vi "show_plot.vi"(6 "plot_id":i32, 8 "autoscale":bool, 9 "show_plot":bool, 11 "XYGraph Refnum":refnum<vi>) -> (0 "done":bool)   [LabVIEW 2025]
uses:
  305b2933-337f-4dbb-963a-25d37b027f8a.vi
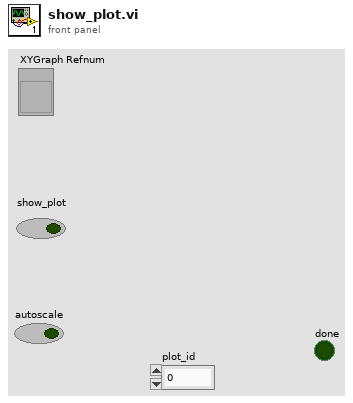
[diagram p1: front panel]
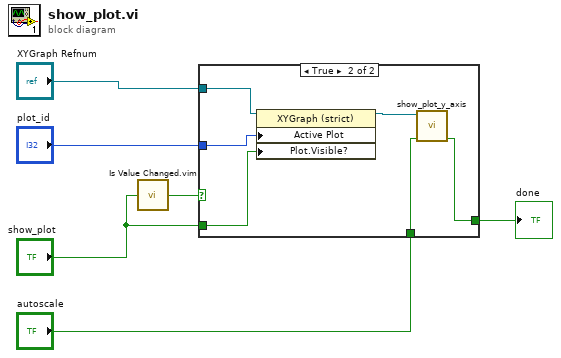
[diagram p0: block diagram]
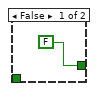
[diagram p2: hidden frame]
diagram:
  n1 = call "Is Value Changed.vim"("value"="show_plot") -> ("changed or first call?"=w6:bool)
  n2 = case shown="True" w6 {
    tunnel: "show_plot" -> [_ w11]
    tunnel: "XYGraph Refnum" -> [_ w13]
    tunnel: "plot_id" -> [_ w12]
    tunnel: [FALSE w9] -> w2
    tunnel: "autoscale" -> [_ w8]
    frame False {
    }
    frame True {
      n3 = property on="Property Node" class="XYGraph (strict)"(reference=w13, "Active Plot"=w12, "Plot.Visible?"=w11) -> (reference out=w10:refnum<vi>)  [unwired: 1 in, 1 out]
      n4 = call "show_plot_y_axis.vi"("autoscale"=w8, "plot_ref_in"=w10) -> ("done"=w9:bool)  [unwired: 8 in, 1 out]
    }
  }
  "done" <- w2
